vi "overlay oval ajg.vi"(2 "xy coords":cluster{"X Target":sgl, "Y Target":sgl}, 3 "Circle R":i32) -> (0 "Bounding Rectangle":T1)   [LabVIEW 2013]
panel:
  out "x":i32
  out "y":i32
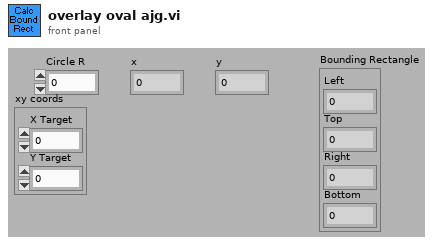
[diagram p1: front panel]
types:
  T1 = cluster{"Left":i32, "Top":i32, "Right":i32, "Bottom":i32}
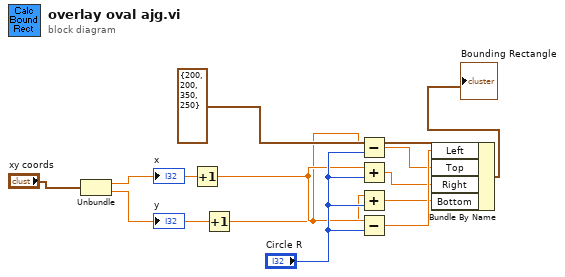
[diagram p0: block diagram]
diagram:
  n1 = Unbundle("xy coords") -> ("X Target"=w2:sgl, "Y Target"=w1:sgl)
  "y" <- w1
  "x" <- w2
  n2 = Increment(x=w2) -> (x+1=w5:sgl)
  n3 = Increment(x=w1) -> (x+1=w4:sgl)
  n4 = Subtract(x=w4, y="Circle R") -> (x-y=w7:sgl)
  n5 = Add(x=w5, y="Circle R") -> (x+y=w8:sgl)
  n6 = Add(x=w4, y="Circle R") -> (x+y=w9:sgl)
  n7 = Subtract(x=w5, y="Circle R") -> (x-y=w10:sgl)
  n8 = Bundle By Name(cluster=T1 {"Left"=200, "Top"=200, "Right"=350, "Bottom"=250} ("Bounding Rectangle"), "Left"=w10, "Top"=w7, "Right"=w8, "Bottom"=w9) -> (→"Bounding Rectangle":T1)
